vi "Update Addon To Latest Version.vi"(8 "error in (no error)":errorcluster, 11 "Device Item Ref in":T1 format="%.0x") -> (0 "error out":errorcluster, 3 "Device Item Ref out":T1 format="%.0x")   [LabVIEW 2019, in "Instrument Addon System Explorer.lvlib"]
uses:
  Instrument Addon System Explorer.lvlib
  <vilib>/NI VeriStand/Custom Device Tools/Custom Device Utility Library/Custom Device Utility Library.lvlib
  <vilib>/NI VeriStand/Custom Device Tools/Custom Device Utility Library/NI VeriStand - Search for All Items by GUID.vi
  Shared/Constants.vi
  Shared/Instrument Addon Shared.lvlib
  <vilib>/NI VeriStand/Custom Device API/Custom Device Channel Type.ctl
  <vilib>/NI VeriStand/Custom Device API/Custom Device API.lvlib
  <vilib>/NI VeriStand/Custom Device API/Custom Device Channel.ctl
  NationalInstruments.VeriStand.SystemDefinitionAPI
  <vilib>/NI VeriStand/Custom Device API/Custom Device Item Ref.ctl
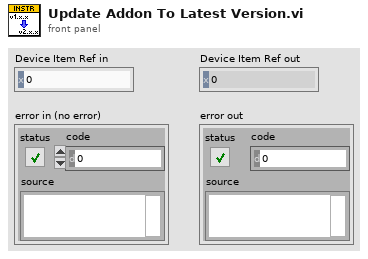
[diagram p1: front panel]
types:
  T1 = typedef "Custom Device API.lvlib/Custom Device Item Ref.ctl" = u64
  T2 = typedef "Custom Device API.lvlib/Custom Device Channel.ctl" = cluster{"Type":T3, "Units":string, "Default Value":dbl, "Faultable":bool, "Scalable":bool}
  T3 = typedef "Custom Device API.lvlib/Custom Device Channel Type.ctl" = enum16{"Input", "Output"}
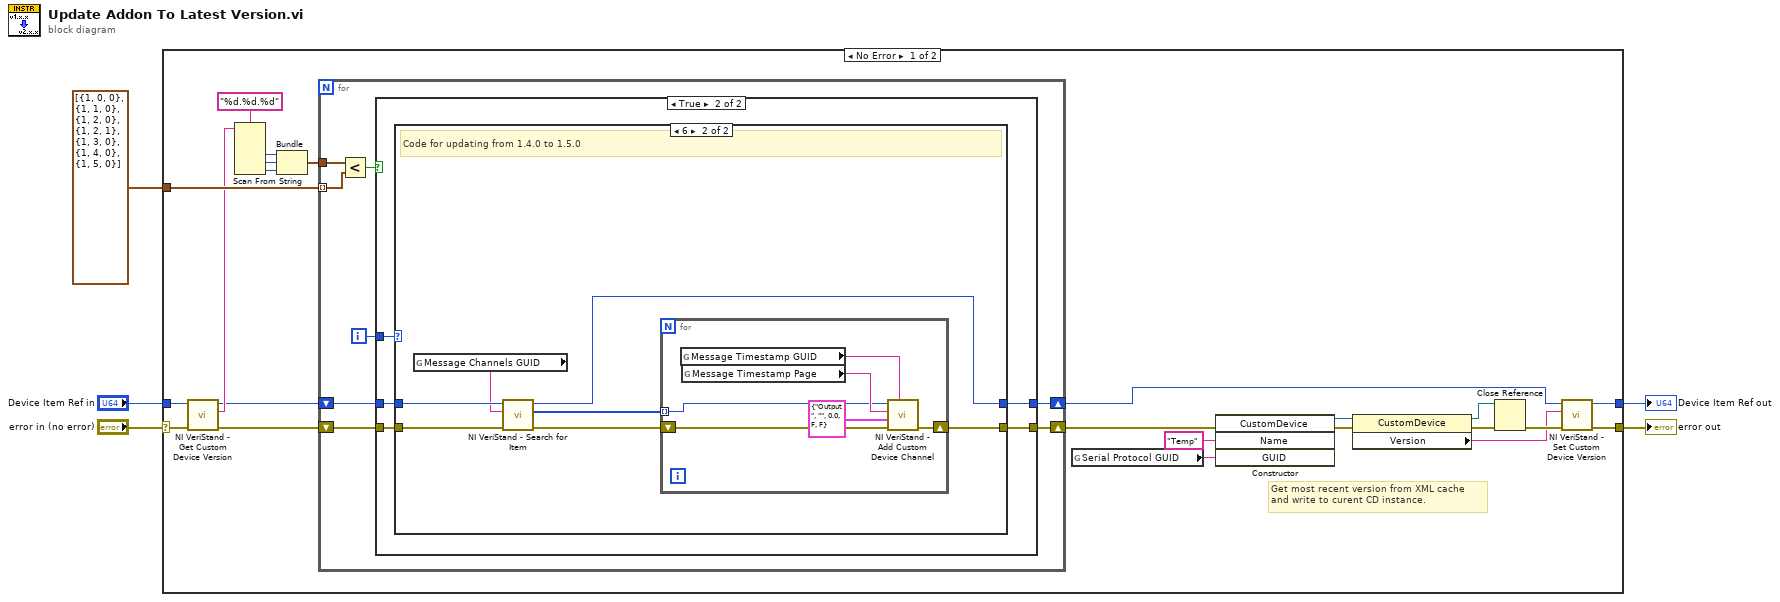
[diagram p0: block diagram]
diagram:
  n1 = case shown="No Error" "error in (no error)" {
    selector: "error in (no error)" -> [w11 w60]
    tunnel: [w20 w60] -> w4
    tunnel: "Device Item Ref in" -> [w10 w59]
    tunnel: [w21 w59] -> w5
    tunnel: cluster{i32, i32, i32}[] [{1, 0, 0}, {1, 1, 0}, {1, 2, 0}, {1, 2, 1}, {1, 3, 0}, {1, 4, 0}, {1, 5, 0}] -> [w28 _]
    frame No Error {
      # "Get most recent version from XML cache\nand write to curent CD instance."
      n2 = call <vilib>:"NI VeriStand - Get Custom Device Version.vi"("error in (no error)"=w11, "Device Ref in"=w10) -> ("error out"=w7:errorcluster, "Value"=w14:string, "Device Ref out"=w6:T1)  [unwired: 7 in]
      n3 = Scan From String(format string="%d.%d.%d", input string=w14) -> (output 1=w13:i32, output 2=w12:i32, output 3=w15:i32)  [unwired: 5 in, 3 out]
      n4 = Bundle(w13, w12, w15) -> (w8:cluster{i32, i32, i32})  [unwired: 1 in]
      n5 = for {
        shift-right: [w35] -> w19
        shift-left: w7 -> [w30]
        shift-right: [w34] -> w18
        shift-left: w6 -> [w29]
        tunnel: w28 -> [w31] mode=indexing
        tunnel: w8 -> [w32]
        i -> [w33]
        n6 = Less?(x=w32, y=w31) -> (x < y?=w36:bool)
        n7 = case shown="True" w36 {
          tunnel: w30 -> [w38 w43]
          tunnel: [w38 w42] -> w35
          tunnel: w29 -> [w37 w39]
          tunnel: [w37 w40] -> w34
          tunnel: w33 -> [_ w41]
          frame False {
          }
          frame True {
            n8 = case shown="6" w41 {
              tunnel: w43 -> [w45 w51]
              tunnel: [w45 w46] -> w42
              tunnel: [w44 w47] -> w40
              tunnel: w39 -> [w44 w52]
              frame Default {
              }
              frame 6 {
                # "Code for updating from 1.4.0 to 1.5.0"
                n9 = global read "Constants.vi" "Message Channels GUID"() -> (w50:string)
                n10 = call-poly <vilib>:"NI VeriStand - Search for Item.vi"("error in"=w51, "Item GUID"=w50, "Section Ref in"=w52) -> ("error out"=w49:errorcluster, "Item Refs"=w48:T1[], "Section Ref out"=w47:T1)  [unwired: 5 in, 1 out]
                n11 = for {
                  tunnel: w48 -> [w53] mode=indexing
                  shift-right: [w54] -> w46
                  shift-left: w49 -> [w55]
                  n12 = global read "Constants.vi" "Message Timestamp GUID"() -> (w57:string)
                  n13 = global read "Constants.vi" "Message Timestamp Page"() -> (w58:string)
                  n14 = call <vilib>:"NI VeriStand - Add Custom Device Channel.vi"("GUID (Default Channel)"=w57, "error in (no error)"=w55, "Channel"=T2 {"Type"=enum."Output", "Units"="", "Default Value"=0.0, "Faultable"=FALSE, "Scalable"=FALSE}, "Channel Name"=w58, "Parent Ref in"=w53) -> ("error out"=w54:errorcluster)  [unwired: 3 in, 3 out]
                }
              }
            }
          }
        }
      }
      n15 = global read "Constants.vi" "Serial Protocol GUID"() -> (w16:string)
      n16 = constructor class="CustomDevice"(error in=w19, "Name"="Temp", "GUID"=w16) -> (reference out=w27:refnum<k24>, error out=w26:errorcluster)  [unwired: 2 in, 3 out]
      n17 = property class="CustomDevice"(reference=w27, error in=w26) -> (reference out=w24:refnum<k24>, error out=w25:errorcluster, "Version"=w22:string)
      n18 = Close Reference(reference=w24, error in (no error)=w25) -> (error out=w23:errorcluster)
      n19 = call <vilib>:"NI VeriStand - Set Custom Device Version.vi"("error in (no error)"=w23, "Value"=w22, "Device Ref in"=w18) -> ("error out"=w20:errorcluster, "Device Ref out"=w21:T1)  [unwired: 7 in]
    }
    frame Error {
    }
  }
  "Device Item Ref out" <- w5
  "error out" <- w4
